vi "SrvCreate.vi"(11 "error in (no error)":errorcluster) -> (4 "ref out":u64, 15 "error out":errorcluster)   [LabVIEW 2018, in "Snap7.lvlib"]
uses:
  Snap7.lvlib
  windows/lv_snap7.dll
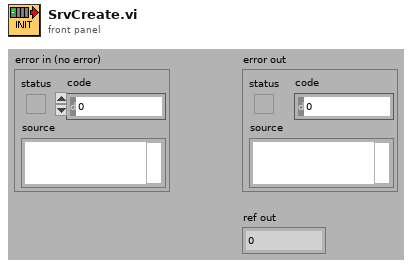
[diagram p1: front panel]
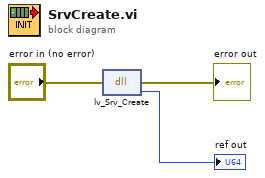
[diagram p0: block diagram]
diagram:
  n1 = dll-call lib="PTH2iabs D项目Feng恒隆项目Labview性能试验台SourcesSnap7libwindowslv_snap7.dll" fn="lv_Srv_Create"(error in="error in (no error)") -> (error out=→"error out":errorcluster, "return type"=→"ref out":u64)  [unwired: 2 in, 1 out]
